vi "Read AI.vi"(8 "error in (no error)":errorcluster, 11 "Refnum in":refnum<k20>) -> (0 "error out":errorcluster, 3 "data":cluster{dbl, dbl, dbl, dbl})   [LabVIEW 2024]
uses:
  <vilib>/Utility/error.llb/Error Cluster From Error Code.vi
  <vilib>/RVI Host/nirviSupport.llb/nirviErrorClusterFromErrorCode.vi
  <vilib>/rvi/errors/niLvFpgaAdjustHostInterfaceError.vi
  <vilib>/rvi/interface/nirviMethod/nirviMethod.xnode
  <vilib>/rvi/interface/nirviReadWriteControl/nirviReadWriteControl.xnode
  <vilib>/rvi/interface/nirviMethod/StockFPGA_InlinedMethodWaitForSingleIRQ.vi
  <vilib>/FPGAPlugInAG/Dynamic/niLvFpga_WaitOnIrq_Dynamic.vi
  <vilib>/FPGAPlugInAG/Dynamic/niLvFpga_AcknowledgeIrq_Dynamic.vi
  NiFpgaLv.dll
  <vilib>/rvi/interface/Simulation/niFpgaSimulationCallBeginRW.vi
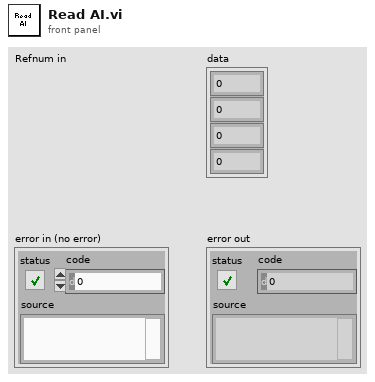
[diagram p1: front panel]
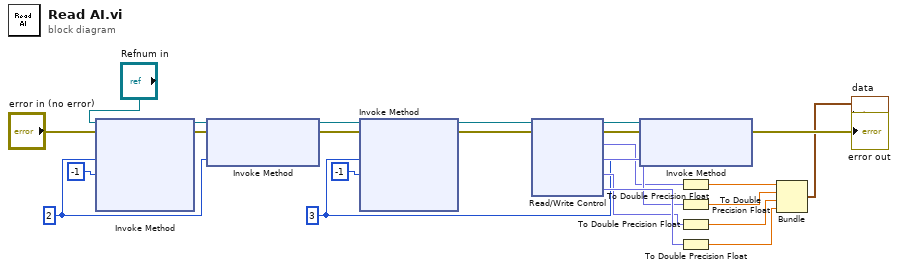
[diagram p0: block diagram]
diagram:
  w6 = 3 ("IRQ Number(s)")
  w3 = 2 ("IRQ Number(s)")
  n1 = xnode "Invoke Method"("FPGA VI Reference In"="Refnum in", "error in"="error in (no error)", "IRQ Number(s)"=w3, "Timeout (ms)"=-1) -> ("FPGA VI Reference Out"=w2:refnum<k20>, "error out"=w1:errorcluster)  [unwired: 2 out]
  n2 = xnode "Invoke Method"("FPGA VI Reference In"=w2, "error in"=w1, "IRQ Number(s)"=w3) -> ("FPGA VI Reference Out"=w8:refnum<k20>, "error out"=w9:errorcluster)
  n3 = xnode "Invoke Method"("FPGA VI Reference In"=w8, "error in"=w9, "IRQ Number(s)"=w6, "Timeout (ms)"=-1) -> ("FPGA VI Reference Out"=w10:refnum<k20>, "error out"=w11:errorcluster)  [unwired: 2 out]
  n4 = xnode "Read/Write Control"("FPGA VI Reference In"=w10, "error in"=w11) -> ("FPGA VI Reference Out"=w12:refnum<k20>, "error out"=w13:errorcluster, "Mod1/AI0"=w20:fxp<+/-,17,5>, "Mod1/AI1"=w21:fxp<+/-,17,5>, "Mod1/AI2"=w22:fxp<+/-,17,5>, "Mod1/AI3"=w23:fxp<+/-,17,5>)
  n5 = xnode "Invoke Method"("FPGA VI Reference In"=w12, "error in"=w13, "IRQ Number(s)"=w6) -> ("error out"=→"error out":errorcluster)  [unwired: 1 out]
  n6 = To Double Precision Float(number=w20) -> (double precision float=w14:dbl)
  n7 = To Double Precision Float(number=w21) -> (double precision float=w15:dbl)
  n8 = To Double Precision Float(number=w22) -> (double precision float=w16:dbl)
  n9 = To Double Precision Float(number=w23) -> (double precision float=w17:dbl)
  n10 = Bundle(w14, w15, w16, w17) -> (→"data":cluster{dbl, dbl, dbl, dbl})  [unwired: 1 in]
